vi "DevScripts_DuplicateCDS.vi"() -> ()   [LabVIEW 2024]
panel:
  out "Conditions":string[](array[string])
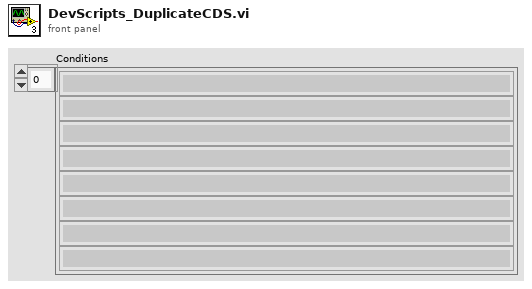
[diagram p1: front panel]
types:
  T1 = enum32{"Conditional Disable Style", "Diagram Disable Style", "Type Specialization Style"}
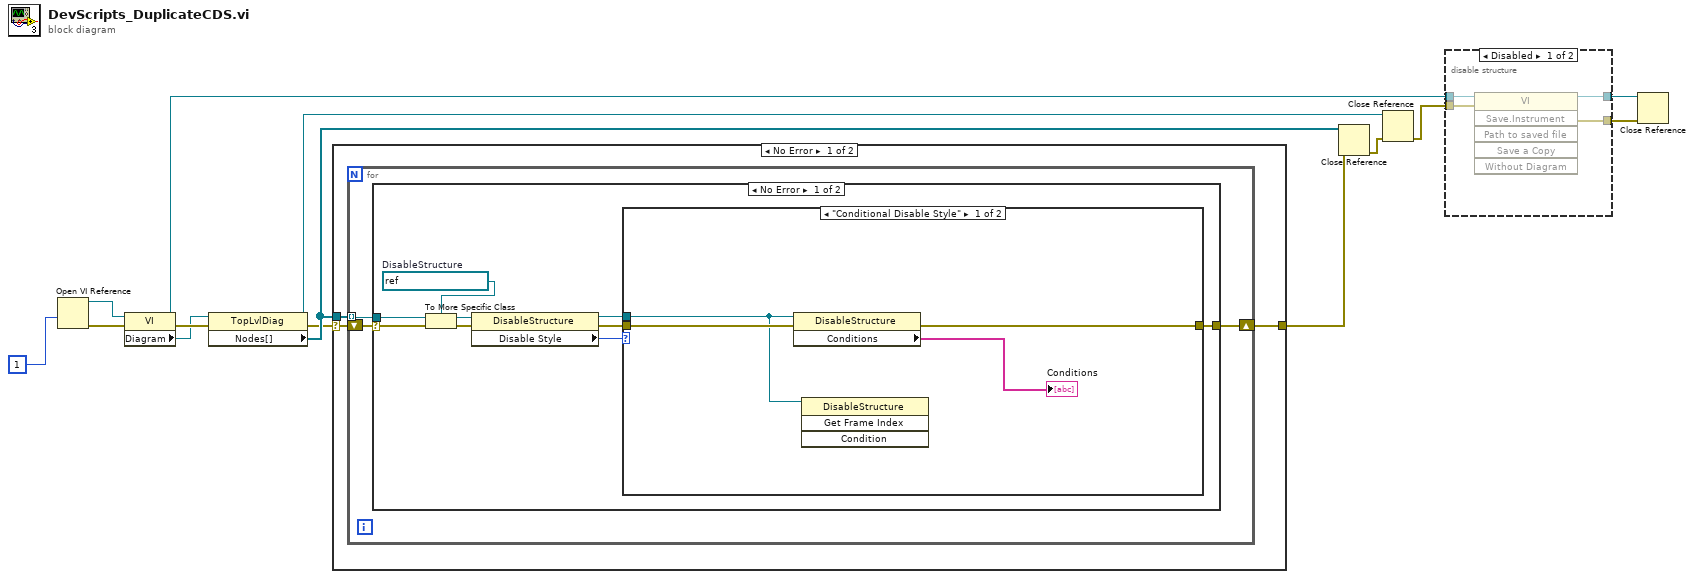
[diagram p0: block diagram]
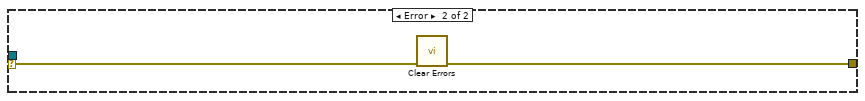
[diagram p4: hidden frame]
diagram:
  n1 = Open VI Reference(options=1) -> (vi reference=w12:refnum<vi>, error out=w13:errorcluster)  [unwired: 5 in]
  n2 = property class="VI"(reference=w12, error in=w13) -> (reference out=w5:refnum<vi>, error out=w11:errorcluster, "Diagram"=w7:refnum<vi>)
  n3 = property class="TopLvlDiag"(reference=w7, error in=w11) -> (reference out=w10:refnum<vi>, error out=w1:errorcluster, "Nodes[]"=w3:refnum<vi>[])
  n4 = case shown="No Error" w1 {
    selector: w1 -> [w15 w37]
    tunnel: w3 -> [w17 _]
    tunnel: [w16 w37] -> w2
    frame No Error {
      n5 = for {
        tunnel: w17 -> [w19] mode=indexing
        shift-right: [w18] -> w16
        shift-left: w15 -> [w20]
        n6 = case shown="No Error" w20 {
          selector: w20 -> [w29 w36]
          tunnel: w19 -> [w27 _]
          tunnel: [w22 w35] -> w18
          frame No Error {
            w26 = refnum<vi> refnum  # DisableStructure
            n7 = To More Specific Class(target class=w26, reference=w27, error in=w29) -> (specific class reference=w25:refnum<vi>, error out=w28:errorcluster)
            n8 = property class="DisableStructure"(reference=w25, error in=w28) -> (reference out=w21:refnum<vi>, error out=w24:errorcluster, "Disable Style"=w23:T1)
            n9 = case shown="\"Conditional Disable Style\"" w23 {
              tunnel: w24 -> [w33 w34]
              tunnel: [w32 w34] -> w22
              tunnel: w21 -> [w30 _]
              frame "Conditional Disable Style" {
                n10 = property class="DisableStructure"(reference=w30, error in=w33) -> (error out=w32:errorcluster, "Conditions"=→"Conditions":string[])  [unwired: 1 out]
                n11 = invoke class="DisableStructure" method="Get Frame Index"(reference=w30) -> ()  [unwired: 3 in, 4 out]
              }
              frame Default {
              }
            }
          }
          frame Error {
            n12 = call <vilib>:"Clear Errors.vi"("error in (no error)"=w36) -> ("error out"=w35:errorcluster)  [unwired: 5 in, 1 out]
          }
        }
      }
    }
    frame Error {
    }
  }
  n13 = Close Reference(reference=w3, error in (no error)=w2) -> (error out=w9:errorcluster)
  n14 = Close Reference(reference=w10, error in (no error)=w9) -> (error out=w8:errorcluster)
  n15 = disable-structure shown="Disabled" {
    disable-tunnel: w8 -> [w41 w43]
    disable-tunnel: [w40 w43] -> w6
    disable-tunnel: w5 -> [w39 w42]
    disable-tunnel: [w38 w42] -> w4
    frame Disabled {
      n16 = invoke class="VI" method="Save.Instrument"(reference=w39, error in=w41) -> (reference out=w38:refnum<vi>, error out=w40:errorcluster)  [unwired: 4 in, 4 out]
    }
    frame Enabled {
    }
  }
  n17 = Close Reference(reference=w4, error in (no error)=w6) -> ()  [unwired: 1 out]
